vi "Pre Launch Init.vi"(11 "TEC Controller in":refnum<class "TEC Controller.lvclass">) -> (0 "error out":errorcluster, 3 "TEC Controller out":refnum<class "TEC Controller.lvclass">)   [LabVIEW 2014, in "Humidifier Test Lib.lvlib" / "TEC Controller.lvclass"]
doc: "(<B>Filename</B>: Actor Framework.lvlib:Actor.lvclass:Pre Launch Init.vi)\n\nDefines behavior that occurs after the Launch Nested Actor method is invoked but before the actor's Actor Core method begins running.\n\nBy default, this method does nothing. A descendant class may override it to define behavior."
uses:
  TEC Controller.lvclass
  reusable/Session APIs/File Access/Config Data/Config Data.lvclass
  reusable/Session APIs/File Access/Config Data/Config Data.lvclass/Config Data.ctl
  TEC Controller.lvclass/TEC Controller.ctl
  reusable/Session APIs/File Access/Config Data/Accessors/Write Cfg Path.vi
  <userlib>/_Session Fwk/Session - Root.lvclass
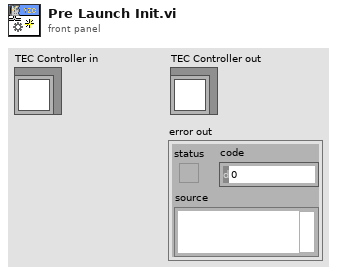
[diagram p1: front panel]
types:
  T1 = typedef "Session - Root.lvclass/Session Handle.ctl" = refnum<data-value>
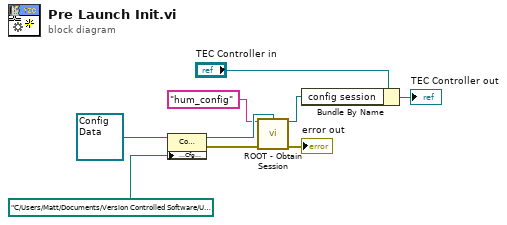
[diagram p0: block diagram]
diagram:
  n1 = property class="Config Data"(reference=refnum<class "Config Data.lvclass"> refnum ("Config Data"), "Accessors:Cfg Path"=path "C:/Users/Matt/Documents/Version Controlled Software/UK Met/Humidifier Test/Controller/humidifier.ini" ("Cfg Path")) -> (reference out=w8:refnum<class "Config Data.lvclass">, error out=w6:errorcluster)  [unwired: 1 in]
  n2 = call <userlib>:"ROOT - Obtain Session.vi"("Session Name ()"="hum_config", "OBJ - Session"=w8, "error in (no error)"=w6) -> ("Session Handle"=w3:T1, "error out"=→"error out":errorcluster)  [unwired: 10 in, 1 out]
  n3 = Bundle By Name(cluster="TEC Controller in", "config session"=w3) -> (→"TEC Controller out":refnum<class "TEC Controller.lvclass">)
